vi "LUCS001RT_GPS_RS232_GetU8Data.vi"(1 "N-Bytes":u8[](array[numeric])=[96, 57, 252, 15, 42, 208, 229, 185, 4, 137, 9, 20, 84, 3, 3, 0, 255, 136, 3, 0, 136, 15, 0, 0, 223, 21, 0, 0, 116, 9] format="%02x", 3 "index":i32) -> (0 "U8":u8)   [LabVIEW 2020]
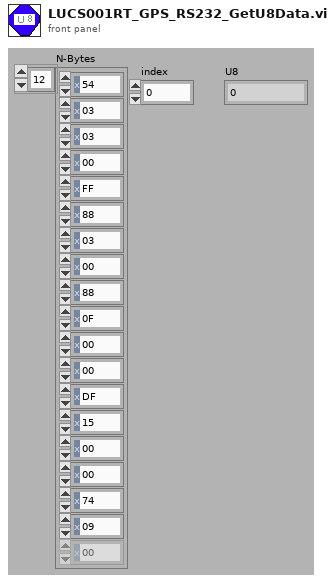
[diagram p1: front panel]
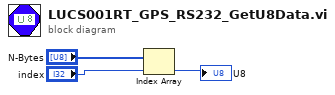
[diagram p0: block diagram]
diagram:
  n1 = Index Array(array="N-Bytes", index="index") -> (element=→"U8":u8)
